vi "Remove empty strings from array.vi"(1 "Array in":string[](array[string])) -> (0 "Array out":string[](array[string]))   [LabVIEW 2013]
doc: "Removes empty strings from an array of strings."
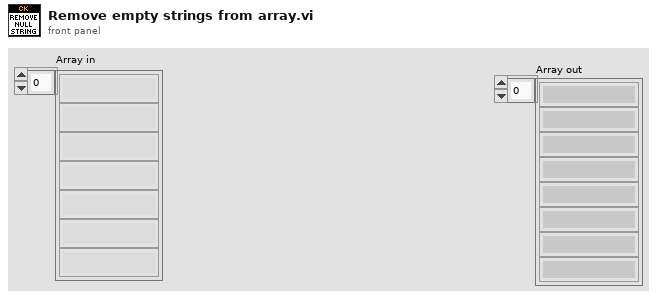
[diagram p1: front panel]
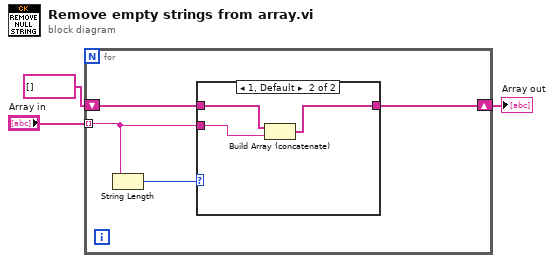
[diagram p0: block diagram]
diagram:
  n1 = for {
    tunnel: "Array in" -> [w6] mode=indexing
    shift-right: [w5] -> w1
    shift-left: string[] [] -> [w4]
    n2 = String Length(string=w6) -> (length=w7:i32)
    n3 = case shown="1, Default" w7 {
      tunnel: w6 -> [_ w11]
      tunnel: [w8 w10] -> w5
      tunnel: w4 -> [w8 w9]
      frame 0 {
      }
      frame 1, Default {
        n4 = Build Array (concatenate)(w9, w11) -> (w10:string[])
      }
    }
  }
  "Array out" <- w1
